vi "test-runner.vi"() -> ()   [LabVIEW 2021]
panel:
  out "Result":u32(colorbox)
  in  "Detail":string
  in  "List of tests":T1(array[cluster])=[{"VI Path"="..\\lib\\SetGetControlValue\\test\\test-SetGetControlValue.vi", "Result"="GOOD\n", "Enabled"=TRUE}, {"VI Path"="..\\lib\\SetGetControlValue\\test\\test-SetGetControlValues.vi", "Result"="GOOD\n", "Enabled"=TRUE}, {"VI Path"="..\\lib\\File\\test\\test-SequentialFileName.vi", "Result"="GOOD\n", "Enabled"=TRUE}, {"VI Path"="..\\lib\\Variant\\test\\test-CoerseNumericTypeFixedPoint.vi", "Result"="", "Enabled"=TRUE}]
  # "Result"
  # "Test/Skip"
  # "Click a test in the left list to show the detailed result. (test number starts from 0)"
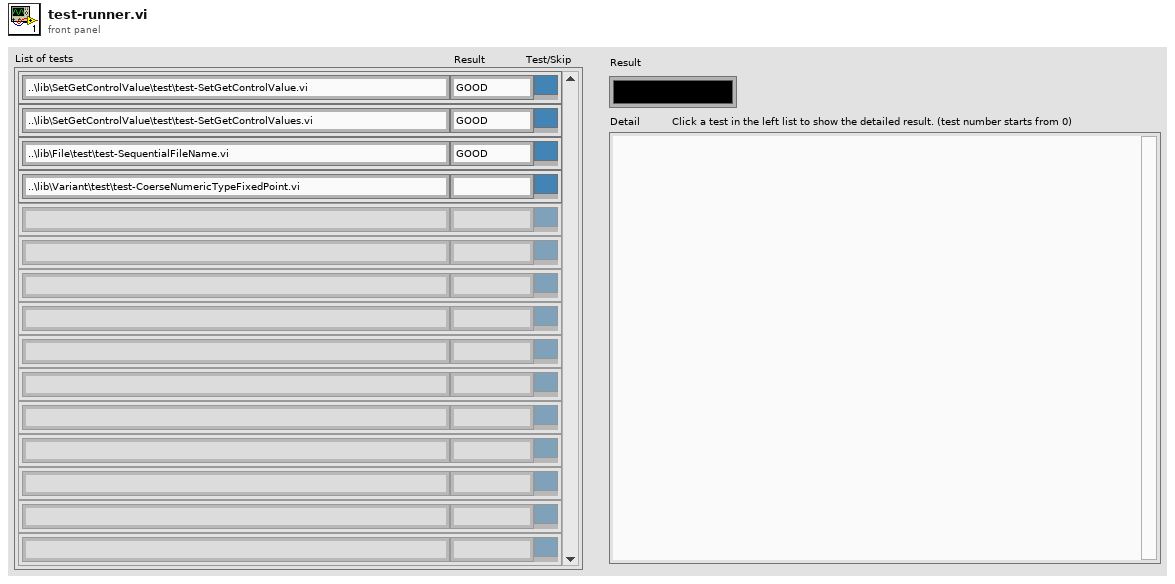
[diagram p1: front panel]
types:
  T1 = cluster{"VI Path":string, "Result":string, "Enabled":bool}[]
  T2 = cluster{"VI Path":string, "Result":string, "Enabled":bool}
  T3 = enum32{"Invalid", "Standard", "Closed", "Hidden", "Minimized", "Maximized"}
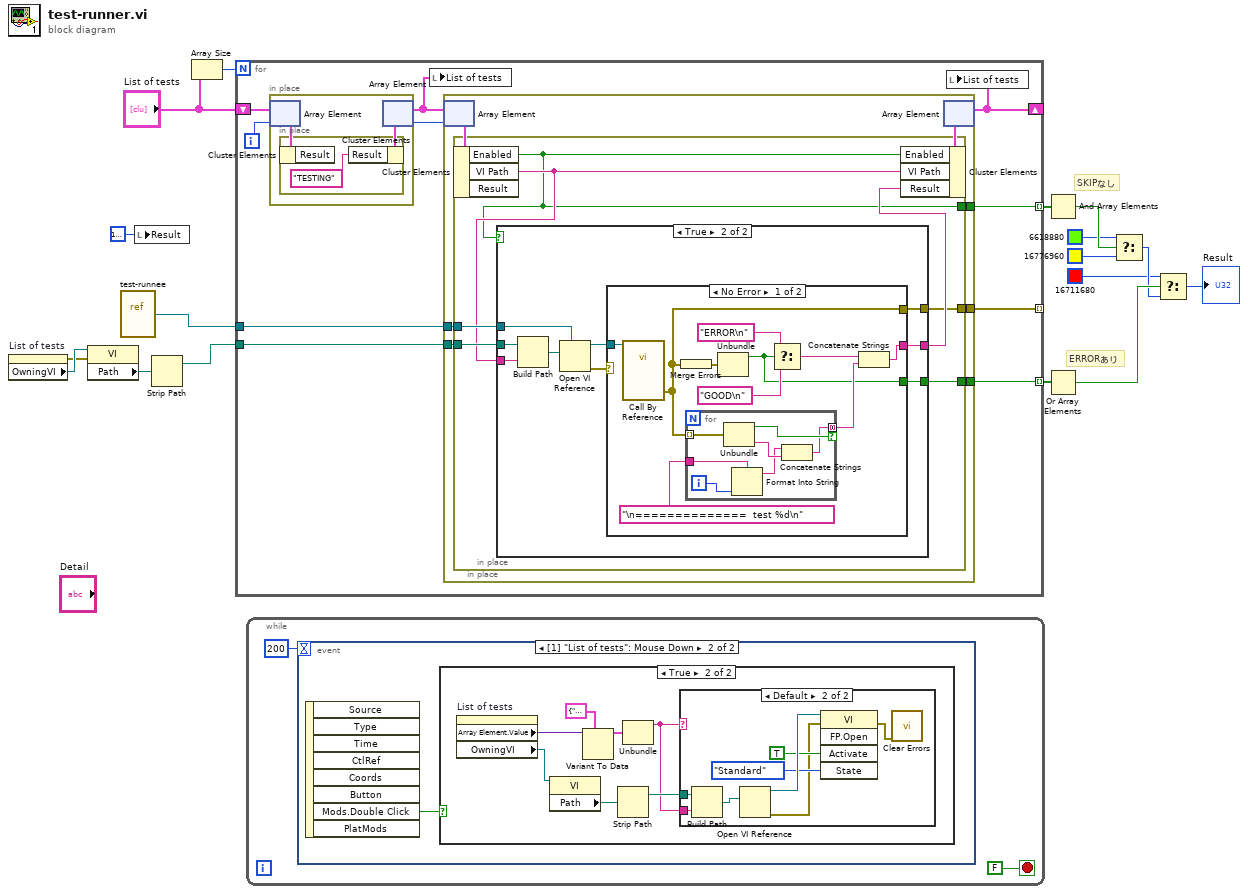
[diagram p0: block diagram]
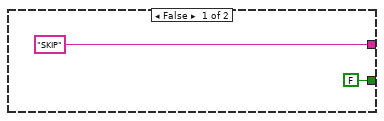
[diagram p2: hidden frame]
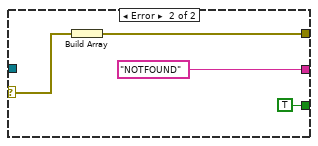
[diagram p3: hidden frame]
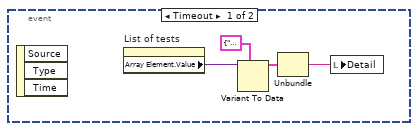
[diagram p4: hidden frame]
diagram:
  # "ERRORあり"
  # "SKIPなし"
  n1 = property on="List of tests" class="Arr (strict)"() -> (error out=w16:errorcluster, "OwningVI"=w17:refnum<vi>)  [unwired: 2 in, 1 out]
  n2 = property class="VI"(reference=w17, error in=w16) -> ("Path"=w15:path)  [unwired: 2 out]
  n3 = vi-ref "test-runnee.vi"() -> (w14:refnum<vi>)
  n4 = local write "Result"(u32 16777222 ("Result")) -> ()
  n5 = Strip Path(path=w15) -> (stripped path=w13:path)  [unwired: 1 out]
  n6 = Array Size(array="List of tests") -> (size(s)=w12:i32)
  n7 = for {
    N: w12 -> [_]
    shift-right: [w21] -> _
    shift-left: "List of tests" -> [w27]
    tunnel: w14 -> [w23]
    tunnel: w13 -> [w22]
    tunnel: [w20] -> _ mode=indexing
    tunnel: [w19] -> w10 mode=indexing
    tunnel: [w18] -> w9 mode=indexing
    i -> [w26]
    n8 = in-place {
      n9 = in-place-array #1(w27, w26) -> (w75:T2)
      n10 = in-place {
        n11 = in-place-cluster #2(w75) -> ()  [unwired: 1 out]
        n12 = in-place-cluster #2("Result"="TESTING") -> (w74:T2)
      }
      n13 = in-place-array #1(w74) -> (w25:T1, w24:i32)
    }
    n14 = local write "List of tests"(w25) -> ()
    n15 = in-place {
      in-place-border: w23 -> [w32]
      in-place-border: w22 -> [w31]
      in-place-border: [w30] -> w20
      in-place-border: [w29] -> w19
      in-place-border: [w28] -> w18
      n16 = in-place-array #3(w25, w24) -> (w34:T2)
      n17 = in-place {
        in-place-border: w32 -> [w41]
        in-place-border: w31 -> [w40]
        in-place-border: [w37] -> w30
        in-place-border: [w36] -> w29
        in-place-border: [w35] -> w28
        n18 = in-place-cluster #4(w34) -> ("Enabled"=w36:bool, "VI Path"=w39:string)  [unwired: 1 out]
        n19 = case shown="True" w36 {
          tunnel: w41 -> [_ w51]
          tunnel: [_ w46] -> w37
          tunnel: w40 -> [_ w50]
          tunnel: w39 -> [_ w49]
          tunnel: ["SKIP" ("error message") w47] -> w38
          tunnel: [FALSE ("status") w44] -> w35
          frame False {
          }
          frame True {
            n20 = Build Path(base path=w50, name or relative path=w49) -> (appended path=w48:path)
            n21 = Open VI Reference(type specifier VI Refnum (for type only)=w51, vi path=w48) -> (vi reference=w52:refnum<vi>, error out=w45:errorcluster)  [unwired: 4 in]
            n22 = case shown="No Error" w45 {
              selector: w45 -> [_ w73]
              tunnel: w52 -> [w62 _]
              tunnel: [w57 "NOTFOUND"] -> w47
              tunnel: [w56 w72] -> w46
              tunnel: [w53 TRUE ("status")] -> w44
              frame No Error {
                n23 = call-by-ref "?"(reference=w62) -> ("errors"=w56:errorcluster[])  [unwired: 12 in, 2 out]
                n24 = Merge Errors(w56) -> (w61:errorcluster)
                n25 = for {
                  tunnel: w56 -> [w69] mode=indexing
                  tunnel: [w67] -> w55 mode=concatenating if=w68
                  tunnel: "\n==============  test %d\n" ("delimiter") -> [w64]
                  i -> [w65]
                  n26 = Unbundle(w69) -> ("status"=w68:bool, "source"=w66:string)  [unwired: 1 out]
                  n27 = Format Into String(format string=w64, w65) -> (resulting string=w63:string)  [unwired: 2 in, 1 out]
                  n28 = Concatenate Strings(w63, w66) -> (w67:string)
                }
                n29 = Unbundle(w61) -> ("status"=w53:bool)  [unwired: 2 out]
                n30 = Select(t="ERROR\n", s=w53, f="GOOD\n") -> (s? t:f=w58:string)
                n31 = Concatenate Strings(w58, w55) -> (w57:string)
              }
              frame Error {
                n32 = Build Array(w73) -> (w72:errorcluster[])
              }
            }
          }
        }
        n33 = in-place-cluster #4("Enabled"=w36, "VI Path"=w39, "Result"=w38) -> (w33:T2)
      }
      n34 = in-place-array #3(w33) -> (w21:T1)  [unwired: 1 out]
    }
    n35 = local write "List of tests"(w21) -> ()
  }
  n36 = while {
    stop <- FALSE stop-if-true
    n37 = event shown="[1] \"List of tests\": Mouse Down" {
      selector: _ -> [_ _]
      dyn-events: _ -> [_ _]
      timeout: 200 -> [_ _]
      event Timeout {
        n38 = event-data() -> ()  [unwired: 1 in, 3 out]
        n39 = property on="List of tests" class="Arr (strict)"() -> ("Array Element.Value"=w81:variant)  [unwired: 2 in, 2 out]
        n40 = Variant To Data(type=cluster{string, string, "Enabled":bool} {"", "", "Enabled"=TRUE}, Variant=w81) -> (data=w80:cluster{string, string, "Enabled":bool})  [unwired: 1 in, 1 out]
        n41 = Unbundle(w80) -> (w79:string)  [unwired: 2 out]
        n42 = local write "Detail"(w79) -> ()
      }
      event "List of tests": Mouse Down {
        n43 = event-data() -> ("Mods.Double Click"=w83:bool)  [unwired: 1 in, 7 out]
        n44 = case shown="True" w83 {
          frame False {
          }
          frame True {
            n45 = property on="List of tests" class="Arr (strict)"() -> ("Array Element.Value"=w88:variant, "OwningVI"=w87:refnum<vi>)  [unwired: 2 in, 2 out]
            n46 = property class="VI"(reference=w87) -> ("Path"=w86:path)  [unwired: 1 in, 2 out]
            n47 = Variant To Data(type=cluster{string, string, "Enabled":bool} {"", "", "Enabled"=TRUE}, Variant=w88) -> (data=w89:cluster{string, string, "Enabled":bool})  [unwired: 1 in, 1 out]
            n48 = Strip Path(path=w86) -> (stripped path=w85:path)  [unwired: 1 out]
            n49 = Unbundle(w89) -> (w84:string)  [unwired: 2 out]
            n50 = case shown="Default" w84 {
              tunnel: w85 -> [_ w98]
              tunnel: w84 -> [_ w97]
              frame "" {
              }
              frame Default {
                n51 = Build Path(base path=w98, name or relative path=w97) -> (appended path=w96:path)
                n52 = Open VI Reference(vi path=w96) -> (vi reference=w95:refnum<vi>, error out=w92:errorcluster)  [unwired: 5 in]
                n53 = invoke class="VI" method="FP.Open"(reference=w95, error in=w92, "Activate"=TRUE ("Activate?"), "State"=T3."Standard" ("Front Panel Window:State")) -> (error out=w91:errorcluster)  [unwired: 1 in, 4 out]
                n54 = call <vilib>:"Clear Errors.vi"("error in (no error)"=w91) -> ()  [unwired: 5 in, 2 out]
              }
            }
          }
        }
      }
    }
  }
  n55 = And Array Elements(Boolean array=w10) -> (logical AND=w7:bool)
  n56 = Or Array Elements(Boolean array=w9) -> (logical OR=w8:bool)
  n57 = Select(t=u32 6618880 ("Result"), s=w7, f=u32 16776960 ("Result")) -> (s? t:f=w6:u32)
  n58 = Select(t=u32 16711680 ("Result"), s=w8, f=w6) -> (s? t:f=→"Result":u32)
